vi "INI Write STR.vi"(7 "Section Str":string="Params", 8 "error IN":errorcluster, 9 "Str Val In":string, 10 "Key Str":string, 11 "configuration file path":path=path "D:/3D FIB-SEM Files/Feiss.ini") -> (0 "error out":errorcluster, 3 "file path Out":path)   [LabVIEW 2018]
uses:
  <vilib>/Utility/config.llb/Write Key (String).vi
  <vilib>/Utility/config.llb/NI_LVConfig.lvlib
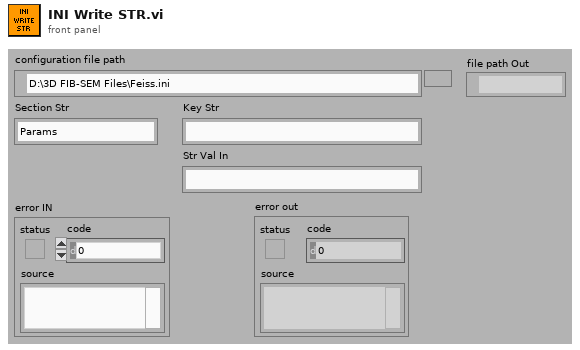
[diagram p1: front panel]
types:
  T1 = typedef "NI_LVConfig.lvlib/Config Data RefNum.ctl" = refnum<k1>
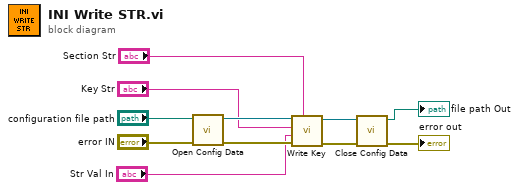
[diagram p0: block diagram]
diagram:
  n1 = call <vilib>:"Open Config Data.vi"("error in (no error)"="error IN", "configuration file path"="configuration file path") -> ("error out"=w10:errorcluster, "refnum"=w11:T1)  [unwired: 7 in, 1 out]
  n2 = call-poly <vilib>:"Write Key.vi"("section"="Section Str", "error in (no error)"=w10, "value"="Str Val In", "key"="Key Str", "refnum"=w11) -> ("error out"=w9:errorcluster, "refnum out"=w8:T1)  [unwired: 4 in, 1 out]
  n3 = call <vilib>:"Close Config Data.vi"("error in (no error)"=w9, "refnum"=w8) -> ("error out"=→"error out":errorcluster, "file path"=→"file path Out":path)  [unwired: 8 in]
